vi "ATSpectrograph_logEvent_timeout.vi"(8 "error in (no error)":errorcluster, 11 "logevent_timeout_Ctl":T1) -> (0 "error out":errorcluster, 2 "function return":i32, 3 "logevent_timeout_Ctl out":T1)   [LabVIEW 2016, in "SALLV_ATSpectrograph.lvlib"]
doc: "int ATSpectrograph_shm_logEvent_timeoutLV(ATSpectrograph_logevent_timeoutLV *logevent_timeout_Ctl );"
uses:
  SALLV_ATSpectrograph.lvlib
  DataTypes/logevent_timeout.ctl
  SALLV_ATSpectrograph.so
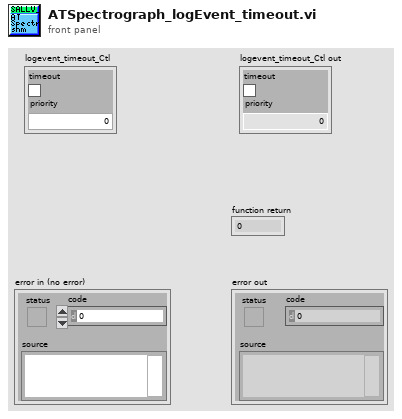
[diagram p1: front panel]
types:
  T1 = typedef "SALLV_ATSpectrograph.lvlib/logevent_timeout.ctl" = cluster{"timeout":bool, "priority":i32}
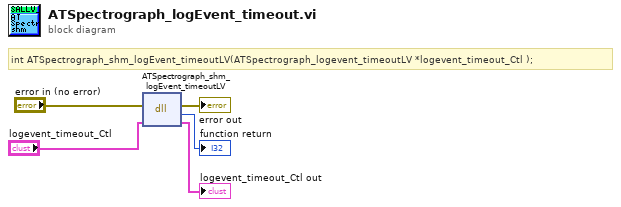
[diagram p0: block diagram]
diagram:
  # "int ATSpectrograph_shm_logEvent_timeoutLV(ATSpectrograph_logevent_timeoutLV *logevent_timeout_Ctl );"
  n1 = dll-call lib="home/harini/TCS/develop/SALLV_ATSpectrograph/SALLV_ATSpectrograph.*" fn="ATSpectrograph_shm_logEvent_timeoutLV"(error in="error in (no error)", "logevent_timeout_Ctl"="logevent_timeout_Ctl") -> (error out=→"error out":errorcluster, →"function return":i32, "logevent_timeout_Ctl"=→"logevent_timeout_Ctl out":T1)  [unwired: 2 in, 1 out]
